vi "LTE_Example.vi"() -> ()   [LabVIEW 2016]
uses:
  Source/SA/RFmxLTE/Typedefs/LTE ModAcc Configuration.ctl
  Source/SA/RFmxLTE/Typedefs/LTE ModAcc Results.ctl
  Source/SA/RFmxLTE/Typedefs/LTE ModAcc Component Carrier Results.ctl
  Source/SA/RFmxInstr/Typedefs/Instrument Configuration.ctl
  Source/Common/Local Oscillator Sharing Mode.ctl
  Source/Common/SA Common Configuration.ctl
  Source/SA/RFmxLTE/Typedefs/LTE Standard Configuration.ctl
  Source/SA/RFmxLTE/Typedefs/LTE Component Carrier Configuration.ctl
  Source/SA/RFmxLTE/RFmxLTE.lvlib
  Source/SA/RFmxInstr/RFmxInstr.lvlib
  Source/Common/Common.lvlib
panel:
  out "error out":errorcluster
  out "ModAcc Results":T1
  in  "Tab Control":enum32{"Common", "Standard", "ACP", "ModAcc"}(tab)
  in  "Resource Name":refnum<k15>="VST"
  in  "Common Configuration":T3={"Center Frequency (Hz)"=3500000000.0, "Reference Level (dBm)"=0.0, "External Attenuation (dB)"=0.0, "Trigger Enabled"=TRUE, "Digital Trigger Source"="PXI_Trig0", "Trigger Delay (s)"=0.0, "Selected Ports"=""} {"Trigger Delay (s)" format="%.2p"; "External Attenuation (dB)" format="%.2f"; "Reference Level (dBm)" format="%.2f"; "Center Frequency (Hz)" format="%.6p"}
  in  "Instrument Configuration":T4={"LO Sharing Mode"=enum."Automatic", "Frequency Reference Source"="PXI_Clk"}
  in  "LTE Standard Configuration":T6={"Link Direction"=1, "Duplex Scheme"=0, "Uplink Downlink Configuration"=0, "Band"=1, "PUSCH Auto Resource Block Detection Enabled"=1, "Auto DMRS Detection Enabled"=1, "Downlink Auto Cell ID Detection Enabled"=0, "Component Carrier Configurations"=[{"Bandwidth (Hz)"=20000000.0, "Cell ID"=0, "PUSCH Modulation Type"=0, "PUSCH Resource Block Offset"=0, "PUSCH Number of Resource Blocks"=-1, "Downlink Test Model"=0}]} {"Downlink Auto Cell ID Detection Enabled" items=["False", "True"]; "Link Direction" items=["Downlink", "Uplink"]; "Auto DMRS Detection Enabled" items=["False", "True"]; "PUSCH Auto Resource Block Detection Enabled" items=["False", "True"]; "Component Carrier Configurations"."Downlink Test Model" items=["TM1.1", "TM1.2", "TM2", "TM 2a", "TM 3.1", "TM 3.2", "TM 3.3", "TM 3.1a"]; "Component Carrier Configurations"."PUSCH Modulation Type" items=["QPSK", "16 QAM", "64 QAM", "256 QAM", "1024 QAM"]; "Component Carrier Configurations"."Bandwidth (Hz)" items=["200.0 k"=200000.0, "1.4 M"=1400000.0, "3.0 M"=3000000.0, "5.0 M"=5000000.0, "10.0 M"=10000000.0, "15.0 M"=15000000.0, "20.0 M"=20000000.0]; "Uplink Downlink Configuration" items=["0", "1", "2", "3", "4", "5", "6"]; "Duplex Scheme" items=["FDD", "TDD", "LAA"]}
  in  "ModAcc Configuration":T8={"Synchronization Mode"=1, "Measurement Offset"=0, "Measurement Length"=1, "EVM Unit"=0, "Averaging Enabled"=0, "Averaging Count"=10} {"Averaging Enabled" items=["Percentage", "dB"]; "EVM Unit" items=["Percentage", "dB"]; "Synchronization Mode" items=["Frame", "Slot", "Marker"]}
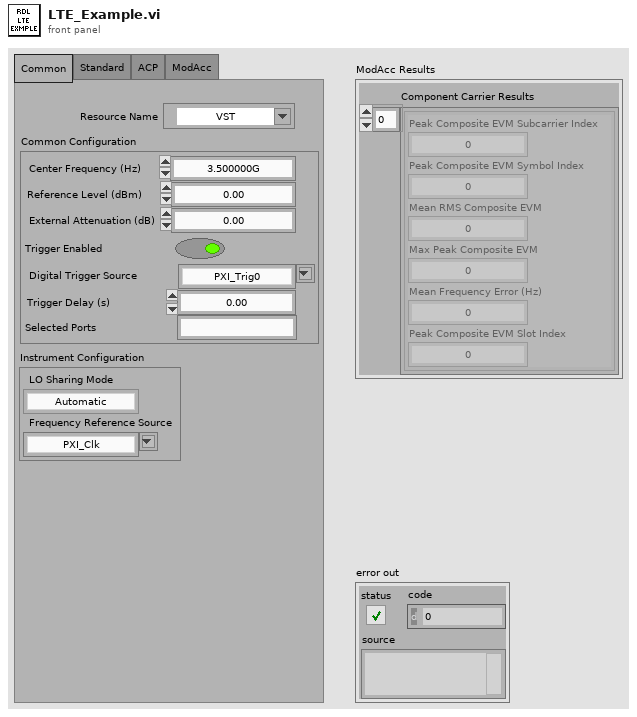
[diagram p1: front panel]
types:
  T1 = typedef "RFmxLTE.lvlib/LTE ModAcc Results.ctl" = cluster{"Component Carrier Results":T2[]}
  T2 = typedef "RFmxLTE.lvlib/LTE ModAcc Component Carrier Results.ctl" = cluster{"Peak Composite EVM Subcarrier Index":i32, "Peak Composite EVM Symbol Index":i32, "Mean RMS Composite EVM":dbl, "Max Peak Composite EVM":dbl, "Mean Frequency Error (Hz)":dbl, "Peak Composite EVM Slot Index":i32}
  T3 = typedef "Common.lvlib/SA Common Configuration.ctl" = cluster{"Center Frequency (Hz)":dbl, "Reference Level (dBm)":dbl, "External Attenuation (dB)":dbl, "Trigger Enabled":bool, "Digital Trigger Source":string, "Trigger Delay (s)":dbl, "Selected Ports":string}
  T4 = typedef "RFmxInstr.lvlib/Instrument Configuration.ctl" = cluster{"LO Sharing Mode":T5, "Frequency Reference Source":string}
  T5 = typedef "Common.lvlib/Local Oscillator Sharing Mode.ctl" = enum16{"Automatic", "None"}
  T6 = typedef "RFmxLTE.lvlib/LTE Standard Configuration.ctl" = cluster{"Link Direction":i32, "Duplex Scheme":i32, "Uplink Downlink Configuration":i32, "Band":i32, "PUSCH Auto Resource Block Detection Enabled":i32, "Auto DMRS Detection Enabled":i32, "Downlink Auto Cell ID Detection Enabled":i32, "Component Carrier Configurations":T7[]}
  T7 = typedef "RFmxLTE.lvlib/LTE Component Carrier Configuration.ctl" = cluster{"Bandwidth (Hz)":dbl, "Cell ID":i32, "PUSCH Modulation Type":i32, "PUSCH Resource Block Offset":i32, "PUSCH Number of Resource Blocks":i32, "Downlink Test Model":i32}
  T8 = typedef "RFmxLTE.lvlib/LTE ModAcc Configuration.ctl" = cluster{"Synchronization Mode":i32, "Measurement Offset":i32, "Measurement Length":i32, "EVM Unit":i32, "Averaging Enabled":i32, "Averaging Count":i32}
  T9 = enum16{"ACP", "CHP", "ModAcc", "OBW", "SEM", "PVT", "SlotPhase", "SlotPower"}[]
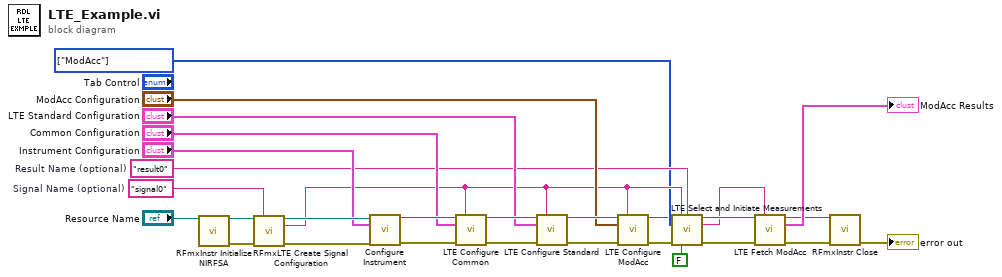
[diagram p0: block diagram]
diagram:
  w9 = T9 [enum."ModAcc"] items=["ACP", "CHP", "ModAcc", "OBW", "SEM", "PVT", "SlotPhase", "SlotPower"] ("Measurements")
  w10 = "result0"  # Result Name (optional)
  w19 = "signal0"  # Signal Name (optional)
  n1 = call <vilib>:"RFmxInstr Initialize NIRFSA.vi"("Resource Name"="Resource Name") -> ("Instrument Handle Out"=w20:refnum<k21>, "error out"=w27:errorcluster)  [unwired: 12 in, 1 out]
  n2 = call <vilib>:"RFmxLTE Create Signal Configuration.vi"("Instrument Handle In"=w20, "Signal Name"=w19, "error in (no error)"=w27) -> ("Instrument Handle Out"=w18:refnum<k21>, "Selector String Out"=w11:string, "error out"=w2:errorcluster)  [unwired: 10 in]
  n3 = call "Configure Instrument.vi"("Instrument Handle In"=w18, "Instrument Configuration"="Instrument Configuration", "error in (no error)"=w2) -> ("Instrument Handle Out"=w17:refnum<k21>, "error out"=w1:errorcluster)  [unwired: 11 in]
  n4 = call "LTE Configure Common.vi"("RFmx Handle In"=w17, "Selector String"=w11, "Common Configuration"="Common Configuration", "error in (no error)"=w1) -> ("RFmx Handle Out"=w29:refnum<k21>, "error out"=w28:errorcluster)  [unwired: 10 in]
  n5 = call "LTE Configure Standard.vi"("RFmx Handle In"=w29, "Selector String"=w11, "LTE Standard Configuration"="LTE Standard Configuration", "error in (no error)"=w28) -> ("RFmx Handle Out"=w25:refnum<k21>, "error out"=w24:errorcluster)  [unwired: 10 in]
  n6 = call "LTE Configure ModAcc.vi"("RFmx Handle In"=w25, "Selector String"=w11, "ModAcc Configuration"="ModAcc Configuration", "error in (no error)"=w24) -> ("RFmx Handle Out"=w6:refnum<k21>, "error out"=w3:errorcluster)  [unwired: 10 in]
  n7 = call "LTE Select and Initiate Measurements.vi"("Instrument Handle In"=w6, "Selector String"=w11, "Result Name"=w10, "Measurements"=w9, "error in (no error)"=w3, "Enable All Traces (F)"=FALSE) -> ("Instrument Handle Out"=w13:refnum<k21>, "Selector String Out"=w8:string, "error out"=w12:errorcluster)  [unwired: 7 in]
  n8 = call "LTE Fetch ModAcc.vi"("RFmx Handle In"=w13, "Selector String"=w8, "error in (no error)"=w12) -> ("RFmx Handle Out"=w5:refnum<k21>, "ModAcc Results"=→"ModAcc Results":T1, "error out"=w4:errorcluster)  [unwired: 10 in]
  n9 = call <vilib>:"RFmxInstr Close.vi"("Instrument Handle In"=w5, "error in (no error)"=w4) -> ("error out"=→"error out":errorcluster)  [unwired: 13 in]
